vi "Call Messenger.vi"(8 "error in (no error)":errorcluster, 11 "System Actor in":refnum<class "System Actor.lvclass">) -> (0 "error out":errorcluster, 2 "Messenger Out":refnum<class "Messenger.lvclass">, 3 "System Actor out":refnum<class "System Actor.lvclass">)   [LabVIEW 2024, in "System Actor.lvclass"]
uses:
  System Actor.lvclass
  Messenger/Messenger/Messenger.lvclass
  System Actor.lvclass/System Actor.ctl
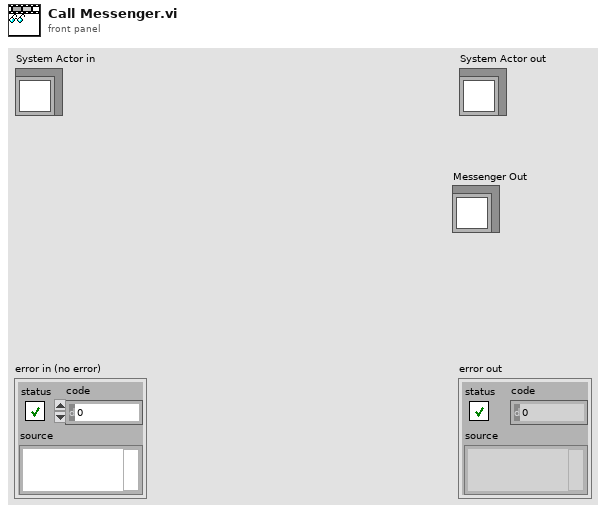
[diagram p1: front panel]
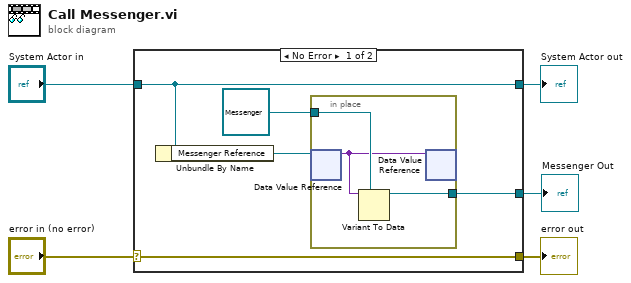
[diagram p0: block diagram]
diagram:
  n1 = case shown="No Error" "error in (no error)" {
    selector: "error in (no error)" -> [w10 w14]
    tunnel: [w10 w14] -> w4
    tunnel: [w9 w15] -> w2
    tunnel: "System Actor in" -> [w9 w15]
    tunnel: [w6 _] -> w1
    frame No Error {
      n2 = Unbundle By Name(w9) -> ("Messenger Reference"=w8:refnum<data-value>)
      n3 = in-place {
        in-place-border: refnum<class "Messenger.lvclass"> refnum ("Messenger Component.lvclass") -> [w13]
        in-place-border: [w11] -> w6
        n4 = in-place-dvr #1(w8) -> (w12:variant)  [unwired: 1 out]
        n5 = Variant To Data(type=w13, Variant=w12) -> (data=w11:refnum<class "Messenger.lvclass">)  [unwired: 1 in, 1 out]
        n6 = in-place-dvr #1(w12) -> ()  [unwired: 2 out]
      }
    }
    frame Error {
    }
  }
  "error out" <- w4
  "System Actor out" <- w2
  "Messenger Out" <- w1
